vi "WebSlider.vi"(8 "Requests to MyWeb (In)":i16, 9 "Read Value":dbl(slide) min=-10.0 max=10.0 step=0.1 scale=-10.0..10.0, 10 "Stored Value (In)":dbl(slide) min=-10.0 max=10.0 step=0.1 scale=-10.0..10.0, 11 "URL":string="myweb.wit.edu/bennetts4/ELEC3800/Lab10/writeVal.php?wrVal=") -> (0 "Requests to MyWeb (Out)":i16, 1 "Path":path, 2 "Body":string, 3 "Header":string)   [LabVIEW 2017]
uses:
  <vilib>/httpClient/LabVIEWHTTPClient.lvlib
panel:
  out "Read Value to Write":dbl
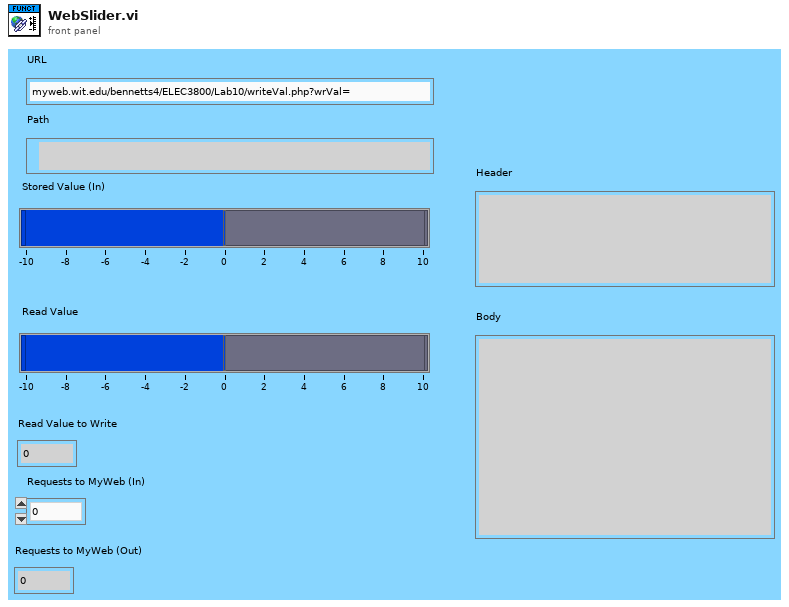
[diagram p1: front panel]
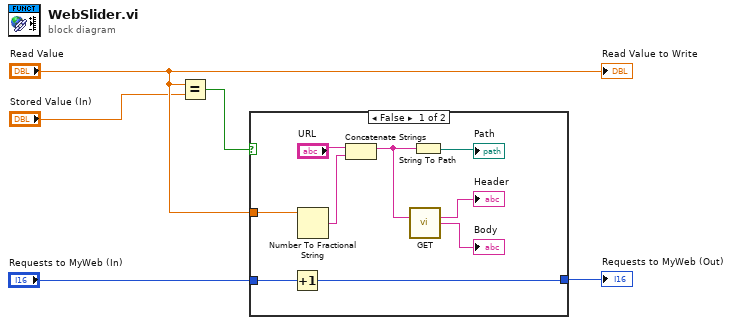
[diagram p0: block diagram]
diagram:
  n1 = Equal?(x="Read Value", y="Stored Value (In)") -> (x = y?=w1:bool)
  n2 = case shown="False" w1 {
    tunnel: "Read Value" -> [w8 _]
    tunnel: "Requests to MyWeb (In)" -> [w7 w15]
    tunnel: [w6 w15] -> w2
    frame False {
      n3 = Increment(x=w7) -> (x+1=w6:i16)
      n4 = Number To Fractional String(number=w8) -> (F-format string=w14:string)  [unwired: 3 in]
      n5 = Concatenate Strings("URL", w14) -> (w11:string)
      n6 = call <vilib>:"GET.vi"("url"=w11) -> ("headers"=→"Header":string, "body"=→"Body":string)  [unwired: 11 in, 2 out]
      n7 = String To Path(string=w11) -> (path=→"Path":path)
    }
    frame True {
    }
  }
  "Requests to MyWeb (Out)" <- w2
  "Read Value to Write" <- "Read Value"
